vi "Example.vi"() -> ()   [LabVIEW 2019, in "ModbusSp.lvclass"]
uses:
  ModbusSp.lvclass
  WriteData.ctl
  ReadData.ctl
panel:
  out "error out 2":errorcluster
  out "read data":T1
  in  "write data":T2
  out "error out":errorcluster
  in  "stop":bool
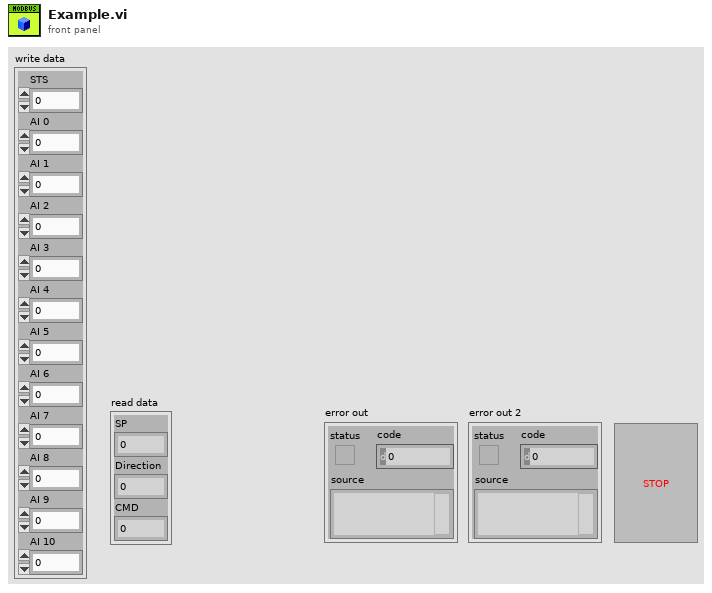
[diagram p1: front panel]
types:
  T1 = typedef "ModbusSp.lvclass/ReadData.ctl" = cluster{"SP":sgl, "Direction":u16, "CMD":u16}
  T2 = typedef "ModbusSp.lvclass/WriteData.ctl" = cluster{"STS":u16, "AI 0":sgl, "AI 1":sgl, "AI 2":sgl, "AI 3":sgl, "AI 4":sgl, "AI 5":sgl, "AI 6":sgl, "AI 7":sgl, "AI 8":sgl, "AI 9":sgl, "AI 10":sgl}
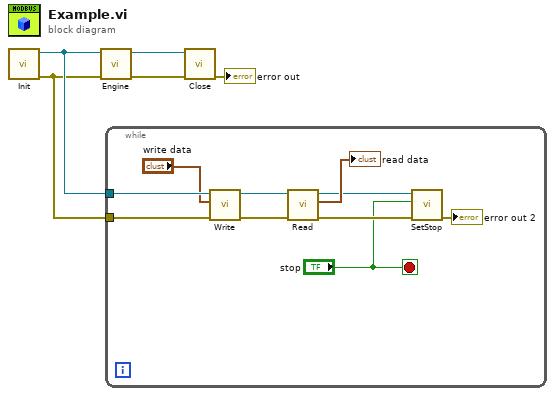
[diagram p0: block diagram]
diagram:
  n1 = call "Init.vi"() -> ("error out"=w1:errorcluster, "ModbusSp out"=w2:refnum<class "ModbusSp.lvclass">)  [unwired: 10 in]
  n2 = call "Engine.vi"("error in (no error)"=w1, "ModbusSp in"=w2) -> ("error out"=w4:errorcluster, "ModbusSp out"=w5:refnum<class "ModbusSp.lvclass">)  [unwired: 8 in]
  n3 = while {
    tunnel: w2 -> [w15]
    tunnel: w1 -> [w14]
    stop <- "stop" stop-if-true
    n4 = call "Write.vi"("error in (no error)"=w14, "write data"="write data", "ModbusSp in"=w15) -> ("error out"=w11:errorcluster, "ModbusSp out"=w12:refnum<class "ModbusSp.lvclass">)  [unwired: 7 in]
    n5 = call "Read.vi"("error in (no error)"=w11, "ModbusSp in"=w12) -> ("error out"=w8:errorcluster, "read data"=→"read data":T1, "ModbusSp out"=w9:refnum<class "ModbusSp.lvclass">)  [unwired: 7 in]
    n6 = call "SetStop.vi"("error in (no error)"=w8, "Value"="stop", "ModbusSp in"=w9) -> ("error out"=→"error out 2":errorcluster)  [unwired: 7 in, 1 out]
  }
  n7 = call "Close.vi"("error in (no error)"=w4, "ModbusSp in"=w5) -> ("error out"=→"error out":errorcluster)  [unwired: 8 in, 1 out]
